vi "Read CtlRef.vi"(8 "error in (no error)":errorcluster, 11 "ListboxDoubleClickMsg in":refnum<class "ListboxDoubleClickMsg.lvclass">) -> (0 "error out":errorcluster, 2 "CtlRef":refnum<vi>, 3 "ListboxDoubleClickMsg out":refnum<class "ListboxDoubleClickMsg.lvclass">)   [LabVIEW 2017, in "ActorEvents.lvlib" / "ListboxDoubleClickMsg.lvclass"]
uses:
  ListboxDoubleClickMsg.lvclass
  ListboxDoubleClickMsg.lvclass/ListboxDoubleClickMsg.ctl
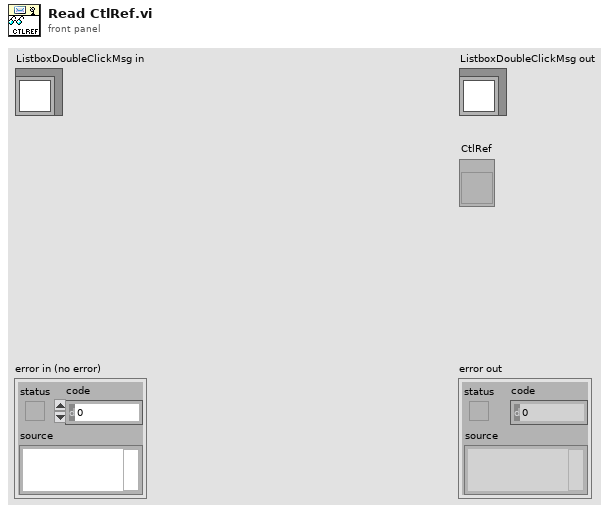
[diagram p1: front panel]
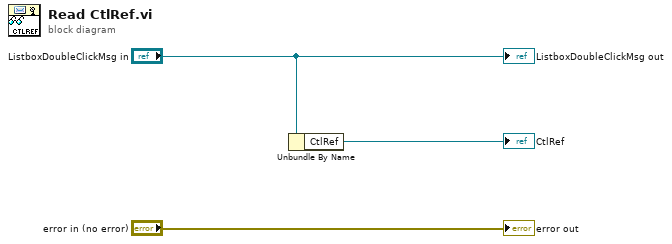
[diagram p0: block diagram]
diagram:
  n1 = Unbundle By Name("ListboxDoubleClickMsg in") -> ("CtlRef"=→"CtlRef":refnum<vi>)
  "error out" <- "error in (no error)"
  "ListboxDoubleClickMsg out" <- "ListboxDoubleClickMsg in"
